vi "Launcher.vi"() -> ()   [LabVIEW 2024]
uses:
  Data Generator_class/Data Generator.lvclass
  <vilib>/Utility/miscctls.llb/LVRectTypeDef.ctl
  Logger_class/Logger.lvclass
  LoggerAdapter_class/LoggerAdapter.lvclass
panel:
  out "Signal Graph":waveform(dbl)(graph)
  in  "Phase":dbl
  in  "Amplitude":dbl
  in  "Frequency":dbl
  in  "Signal Type":T1(ring)
  in  "Stop":bool
  # "750 × 558"
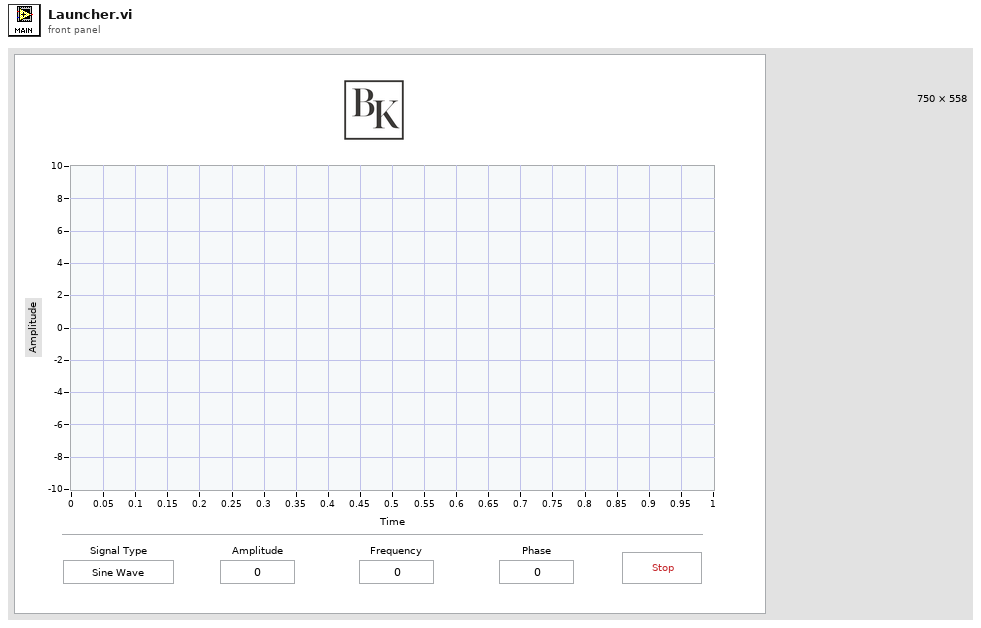
[diagram p1: front panel]
types:
  T1 = enum16{"Sine Wave", "Triangle Wave", "Square Wave", "Sawtooth Wave"}
  T2 = typedef "LVRectTypeDef.ctl" = cluster{"Left":i16, "Top":i16, "Right":i16, "Bottom":i16}
  T3 = typedef "Signal Data.ctl" = cluster{"Signal Out":waveform(dbl)}
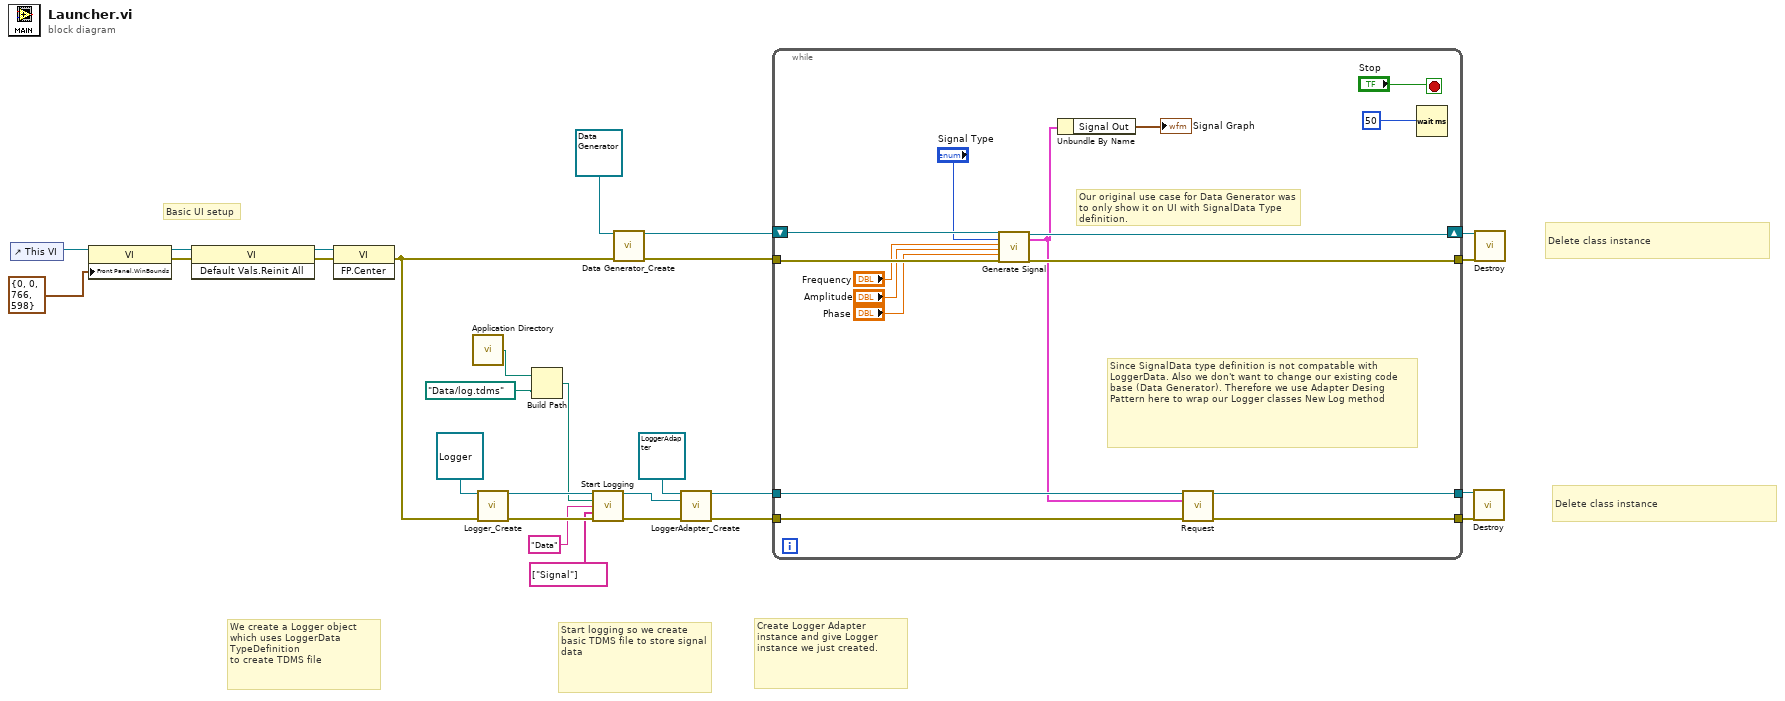
[diagram p0: block diagram]
diagram:
  # "Delete class instance"
  # "Delete class instance"
  # "Create Logger Adapter instance and give Logger instance we just created."
  # "Basic UI setup"
  # "Start logging so we create\nbasic TDMS file to store signal data"
  # "We create a Logger object which uses LoggerData TypeDefinition\nto create TDMS file"
  n1 = control-ref of="This VI"() -> (w22:refnum<vi>)
  n2 = property class="VI"(reference=w22, "Front Panel.WinBounds"=T2 {"Left"=0, "Top"=0, "Right"=766, "Bottom"=598} ("Front Panel Window:Window Bounds")) -> (reference out=w21:refnum<vi>, error out=w20:errorcluster)  [unwired: 1 in]
  n3 = invoke class="VI" method="Default Vals.Reinit All"(reference=w21, error in=w20) -> (reference out=w17:refnum<vi>, error out=w19:errorcluster)  [unwired: 1 in, 1 out]
  n4 = invoke class="VI" method="FP.Center"(reference=w17, error in=w19) -> (error out=w11:errorcluster)  [unwired: 1 in, 2 out]
  n5 = call <vilib>:"Application Directory.vi"() -> ("Application Directory"=w2:path)
  n6 = call "Logger_Create.vi"("reference in"=refnum<class "Logger.lvclass"> refnum ("Logger"), "Error In"=w11) -> ("reference out"=w8:refnum<class "Logger.lvclass">, "Error Out"=w15:errorcluster)  [unwired: 12 in]
  n7 = Build Path(base path=w2, name or relative path=path "Data/log.tdms") -> (appended path=w3:path)
  n8 = call-dynamic "Start Logging.vi"("reference in"=w8, "file path"=w3, "group name"="Data", "channel name"=string[] ["Signal"], "Error In"=w15) -> ("reference out"=w7:refnum<class "Logger.lvclass">, "Error Out"=w6:errorcluster)  [unwired: 9 in]
  n9 = call "Data Generator_Create.vi"("reference in"=refnum<class "Data Generator.lvclass"> refnum ("Data Generator"), "Error In"=w11) -> ("reference out"=w26:refnum<class "Data Generator.lvclass">, "Error Out"=w25:errorcluster)  [unwired: 12 in]
  n10 = call "LoggerAdapter_Create.vi"("reference in"=refnum<class "LoggerAdapter.lvclass"> refnum ("LoggerAdapter"), "Adaptee"=w7, "Error In"=w6) -> ("reference out"=w9:refnum<class "LoggerAdapter.lvclass">, "Error Out"=w10:errorcluster)  [unwired: 11 in]
  n11 = while {
    tunnel: w25 -> [w40]
    tunnel: [w42] -> w23
    shift-right: [w41] -> w24
    shift-left: w26 -> [w39]
    tunnel: w10 -> [w32]
    tunnel: w9 -> [w31]
    tunnel: [w30] -> w5
    tunnel: [w29] -> w4
    stop <- "Stop" stop-if-true
    # "Our original use case for Data Generator was to only show it on UI with SignalData Type definition."
    # "Since SignalData type definition is not compatable with LoggerData. Also we don't want to change our existing code base (Data Generator). Therefore we use Adapter Desing Pattern here to wrap our Logger classes New Log method"
    n12 = call-dynamic "Generate Signal.vi"("reference in"=w39, "signal type"="Signal Type", "frequency"="Frequency", "amplitude"="Amplitude", "phase"="Phase", "Error In"=w40) -> ("reference out"=w41:refnum<class "Data Generator.lvclass">, "Signal Data"=w28:T3, "Error Out"=w42:errorcluster)  [unwired: 11 in]
    n13 = Unbundle By Name(w28) -> ("Signal Out"=→"Signal Graph":waveform(dbl))
    n14 = call-dynamic "Request.vi"("reference in"=w31, "Data"=w28, "Error In"=w32) -> ("reference out"=w30:refnum<class "LoggerAdapter.lvclass">, "Error Out"=w29:errorcluster)  [unwired: 11 in]
    n15 = Wait (ms)(milliseconds to wait=u32 50) -> ()  [unwired: 1 out]
  }
  n16 = call-dynamic "Destroy.vi"("reference in"=w5, "Error In"=w4) -> ()  [unwired: 12 in, 2 out]
  n17 = call-dynamic "Destroy.vi"("reference in"=w24, "Error In"=w23) -> ()  [unwired: 12 in, 2 out]
